vi "Handle error.vi"(8 "error in (no error)":errorcluster, 11 "RxTx in":refnum<class "CCS_RxTx.lvclass">) -> (0 "error out":errorcluster, 3 "RxTx out":refnum<class "CCS_RxTx.lvclass">)   [LabVIEW 2018, in "CCS_RxTx.lvclass"]
uses:
  CCS_RxTx.lvclass
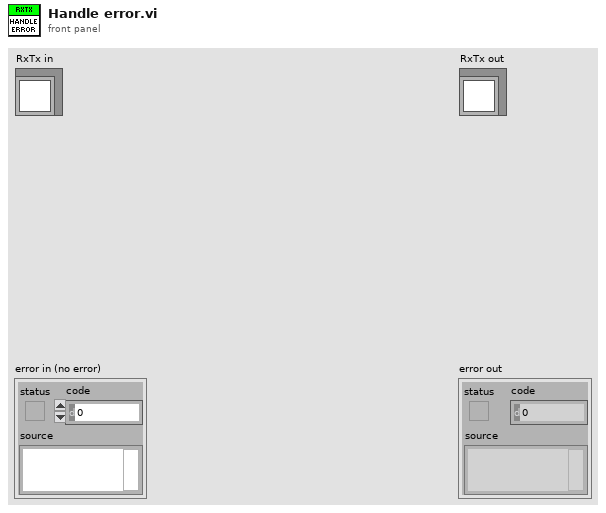
[diagram p1: front panel]
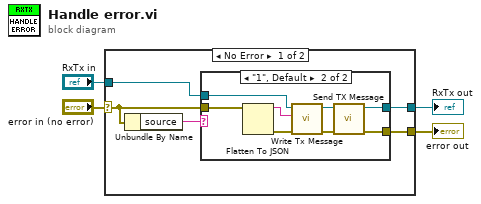
[diagram p0: block diagram]
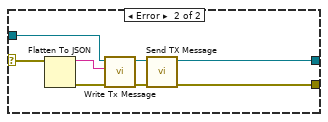
[diagram p3: hidden frame]
diagram:
  n1 = case shown="No Error" "error in (no error)" {
    selector: "error in (no error)" -> [w6 w20]
    tunnel: [w7 w22] -> w3
    tunnel: [w8 w23] -> w1
    tunnel: "RxTx in" -> [w9 w24]
    frame No Error {
      n2 = Unbundle By Name(w6) -> ("source"=w5:string)
      n3 = case shown="\"1\", Default" w5 {
        tunnel: w9 -> [w11 w15]
        tunnel: [w11 w14] -> w8
        tunnel: w6 -> [w10 w12]
        tunnel: [w10 w13] -> w7
        frame "" {
        }
        frame "1", Default {
          n4 = Flatten To JSON(anything=w12) -> (JSON string=w17:string, 11:w16:errorcluster)  [unwired: 2 in]
          n5 = call "Write Tx Message.vi"("error in (no error)"=w16, "Tx Message"=w17, "RxTx in"=w15) -> ("error out"=w18:errorcluster, "RxTx out"=w19:refnum<class "CCS_RxTx.lvclass">)  [unwired: 7 in]
          n6 = call "Send TX Message.vi"("error in (no error)"=w18, "RxTx in"=w19) -> ("error out"=w13:errorcluster, "RxTx out"=w14:refnum<class "CCS_RxTx.lvclass">)  [unwired: 8 in]
        }
      }
    }
    frame Error {
      n7 = Flatten To JSON(anything=w20) -> (JSON string=w25:string, 11:w21:errorcluster)  [unwired: 2 in]
      n8 = call "Write Tx Message.vi"("error in (no error)"=w21, "Tx Message"=w25, "RxTx in"=w24) -> ("error out"=w26:errorcluster, "RxTx out"=w27:refnum<class "CCS_RxTx.lvclass">)  [unwired: 7 in]
      n9 = call "Send TX Message.vi"("error in (no error)"=w26, "RxTx in"=w27) -> ("error out"=w22:errorcluster, "RxTx out"=w23:refnum<class "CCS_RxTx.lvclass">)  [unwired: 8 in]
    }
  }
  "error out" <- w3
  "RxTx out" <- w1
